vi "Constructor.vi"(8 "error in":errorcluster, 9 "Value":T1=enum."NOT_COMPLETED", 10 "Name":string, 11 "ExecutionStatus in":refnum<class "ExecutionStatus.lvclass">) -> (0 "error out":errorcluster, 3 "ExecutionStatus out":refnum<class "ExecutionStatus.lvclass">)   [LabVIEW 2021, in "ProligentXMLGenerator.lvlib" / "ExecutionStatus.lvclass"]
uses:
  ExecutionStatus.lvclass
  ExecutionStatus.lvclass/ExecutionStatus.ctl
  Attribute/Attribute.lvclass
  C:/Projects/proligent-xml-generator-labview/src/ProligentXMLGenerator/Base/Attribute/Attribute.lvclass
  C:/Projects/proligent-xml-generator-labview/src/ProligentXMLGenerator/Base/ExecutionStatus/ExecutionStatus.lvclass
  Value.ctl
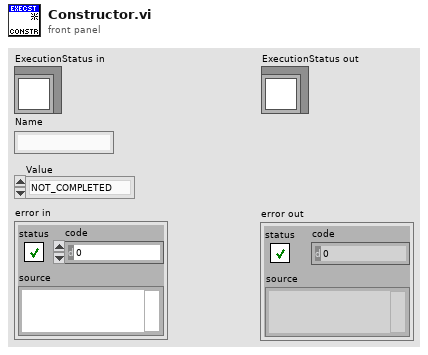
[diagram p1: front panel]
types:
  T1 = typedef "ProligentXMLGenerator.lvlib/ExecutionStatus.lvclass/Value.ctl" = enum16{"PASS", "FAIL", "NOT_COMPLETED", "ABORTED"}
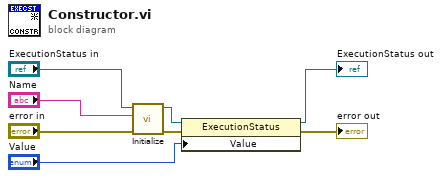
[diagram p0: block diagram]
diagram:
  n1 = call "Initialize.vi"("error in"="error in", "Name"="Name", "Attribute in"="ExecutionStatus in") -> ("error out"=w4:errorcluster, "Attribute out"=w3:refnum<class "ExecutionStatus.lvclass">)  [unwired: 7 in]
  n2 = property on="Property Node" class="ExecutionStatus"(reference=w3, error in=w4, "Value"="Value") -> (reference out=→"ExecutionStatus out":refnum<class "ExecutionStatus.lvclass">, error out=→"error out":errorcluster)
